vi "VI-Hacker.vi"(8 "error in (no error)":errorcluster, 11 "Path to VI (*.vi, *.vit, *.vim)":path) -> (0 "error out":errorcluster)   [LabVIEW 2022 SP3, in "VI-Hacker.lvlib"]
doc: "Unlocks a password protected VI.\n\nCreated by: Ryan Pacini (c) 2023"
uses:
  VI-Hacker.lvlib
panel:
  # "Unlock a Password Protected VI\nCreated by: Ryan Pacini (c) 2023"
  # "Instructions:\n1. Enter path to password protected VI (*.vi)\n2. Run this VI\nNote: A new VI is created, the original source file remains unmodified."
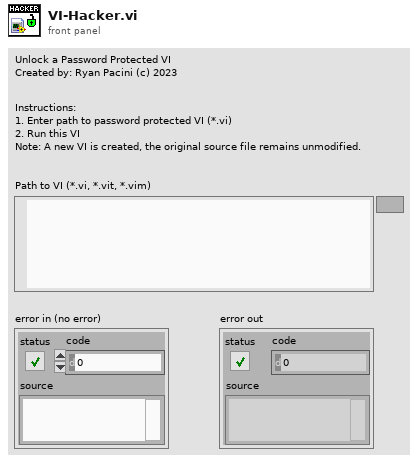
[diagram p1: front panel]
types:
  T1 = cluster{"BLOCK_INFO":cluster{"Int1":u32, "Int2":u32, "Int3":u32, "Offset":u32, "Size":u32}[]}
  T2 = cluster{"Name":string, "Idx":i32, "Data":string, "Offset":u32}
  T3 = enum16{"open", "replace", "create", "open or create", "replace or create", "replace or create with confirmation"}
  T4 = cluster{"vers":i32, "BDPW":i32, "LIBN":i32, "LVSR":i32, "BDHx":i32}
  T5 = cluster{"Version Major":u8, "Pswrd Hashes":cluster{"Pswrd (md5)":string, "Hash1 (md5)":string, "Hash2 (md5)":string}, "Owning Libs (':')":string, "Pswrd Salt (md5)":string, "Diagram (md5)":string, "BDPW Offset":u32, "New BDPW":string}
  T6 = cluster{"Pswrd (md5)":string, "Hash1 (md5)":string, "Hash2 (md5)":string}
  T7 = enum32{"invalid lock state", "Not Locked", "Locked (No Password)", "Password-protected"}
  T8 = cluster{"RSRC_Identifier":u64, "RSRC_Type":u32, "RSRC_Creator":u32, "Info_Offset":u32, "Info_Size":u32, "Data_Offset":u32, "Data_Size":u32}
  T9 = cluster{"Int1":u32, "Int2":u32, "Int3":u32, "Offset":u32, "Size":u32}
  T10 = cluster{"Int1":u32, "Int2":u32, "Int3":u32, "Offset":u32, "Size":u32}[]
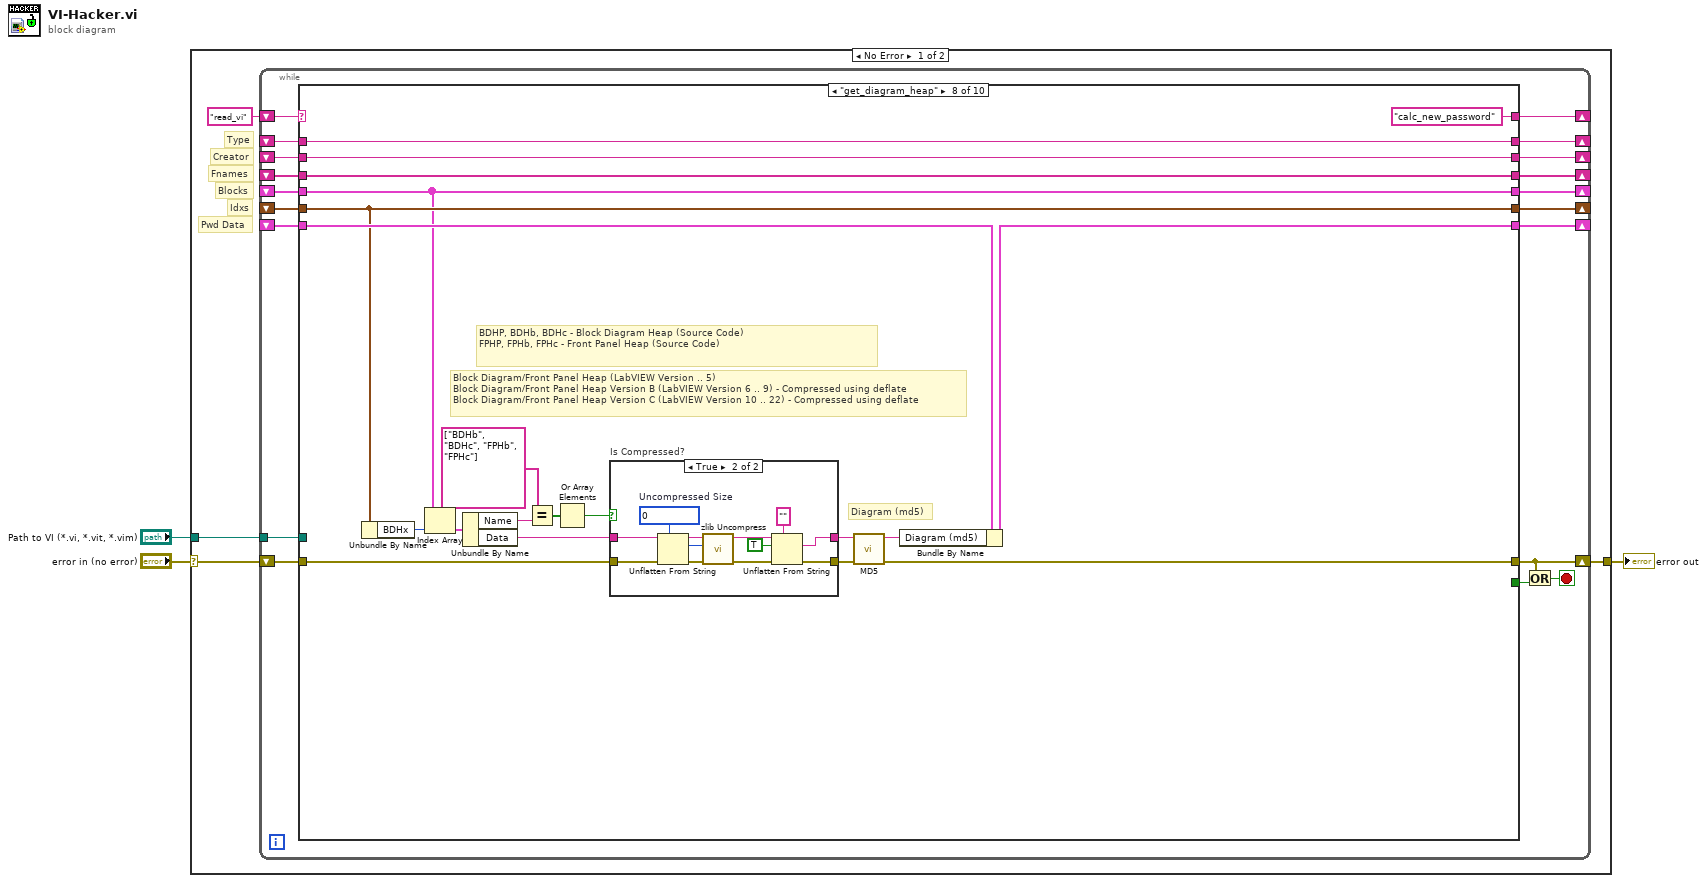
[diagram p0: block diagram]
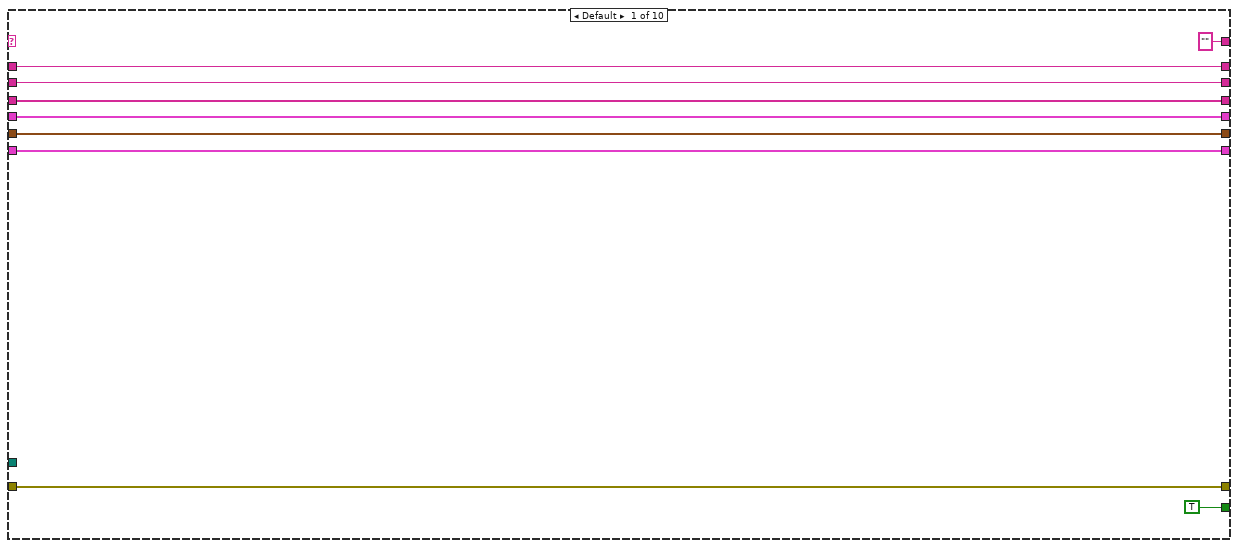
[diagram p2: hidden frame]
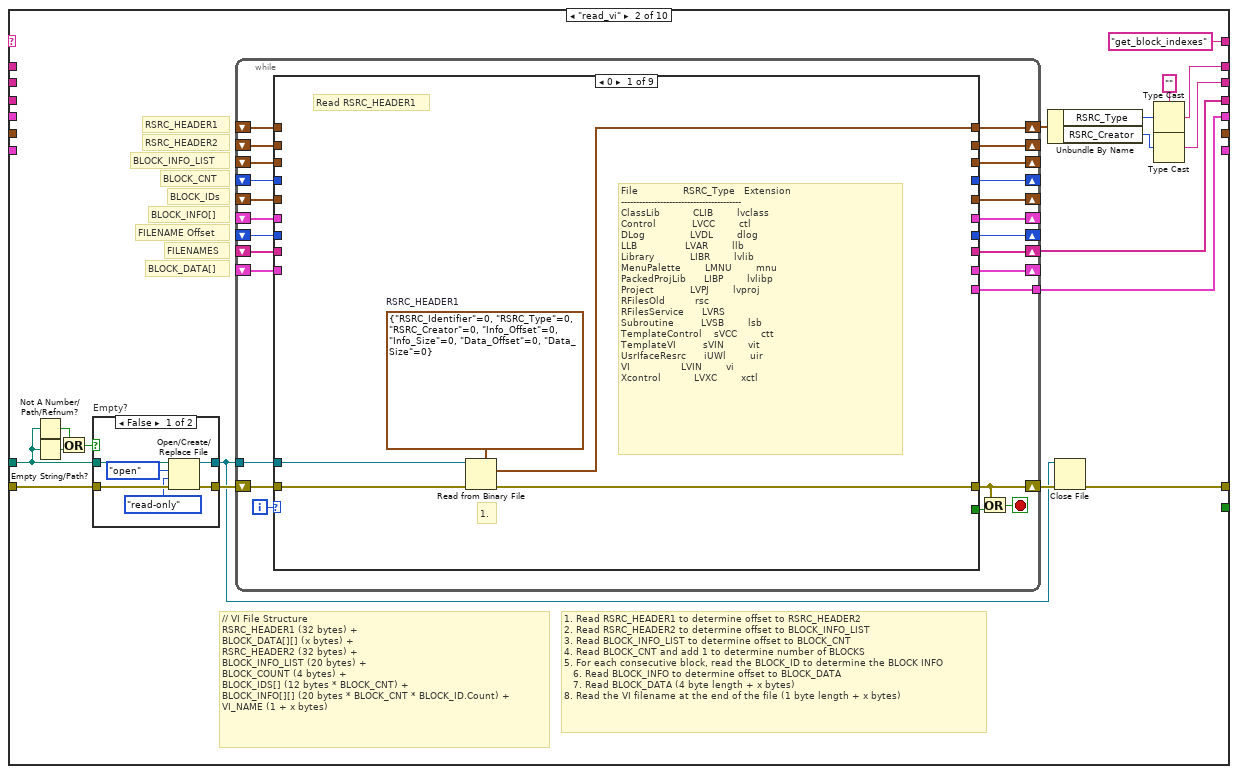
[diagram p3: hidden frame]
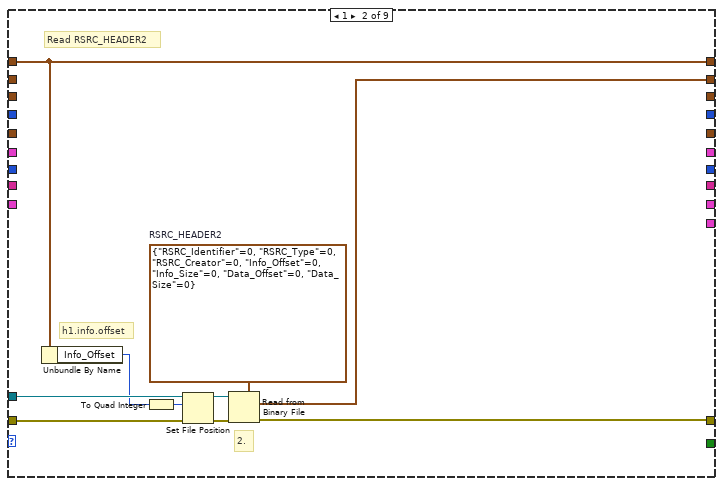
[diagram p4: hidden frame]
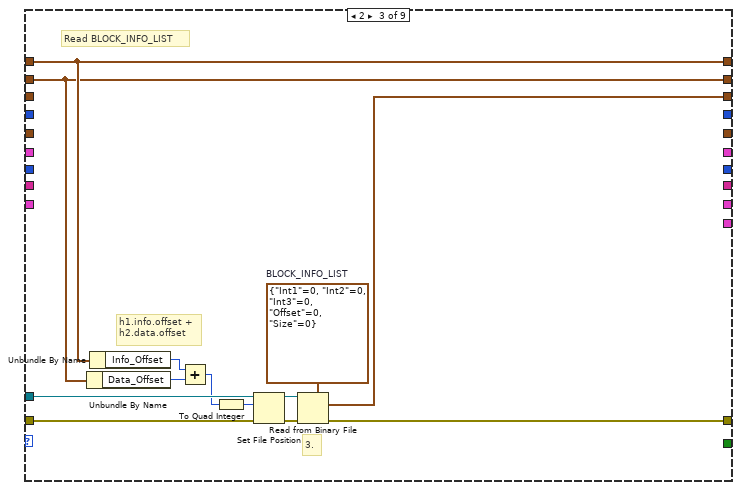
[diagram p5: hidden frame]
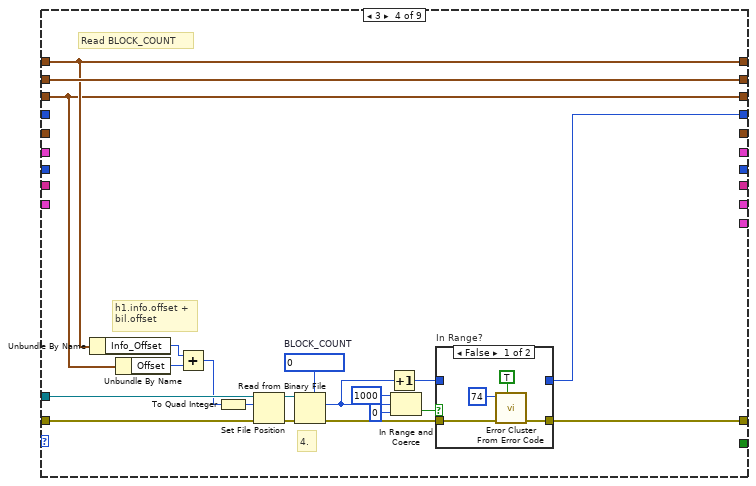
[diagram p6: hidden frame]
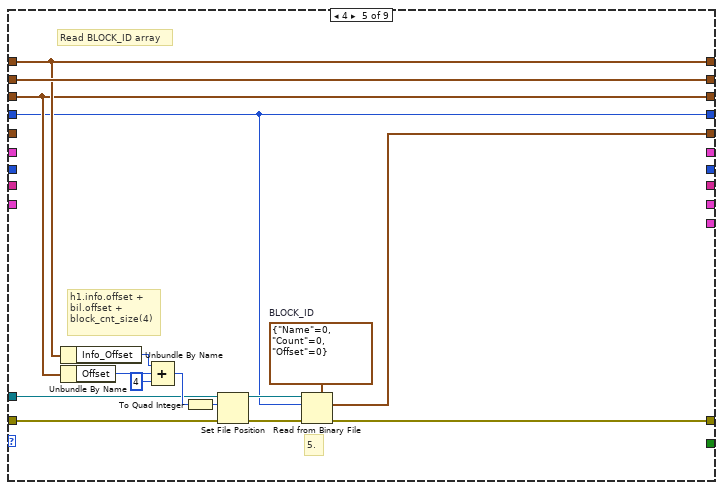
[diagram p8: hidden frame]
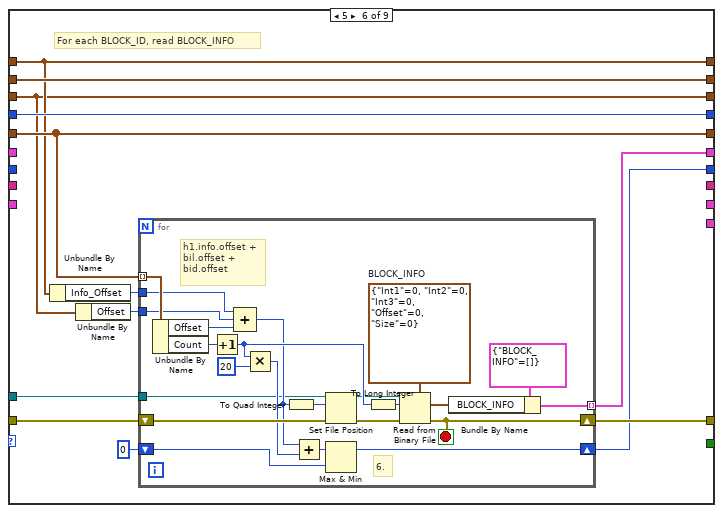
[diagram p9: hidden frame]
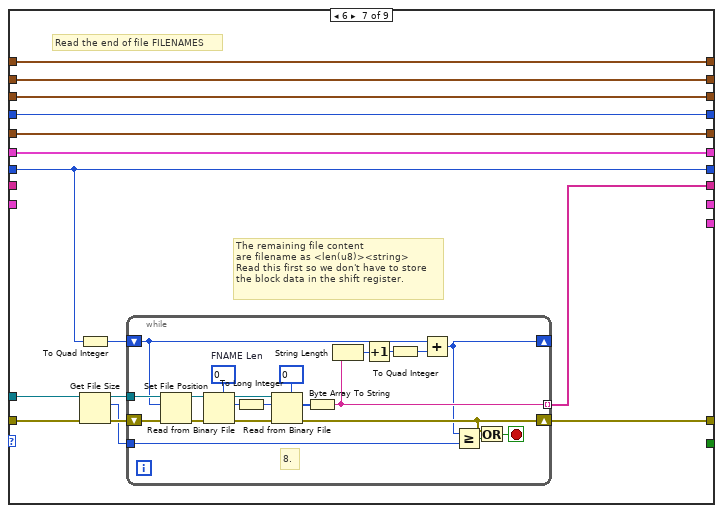
[diagram p10: hidden frame]
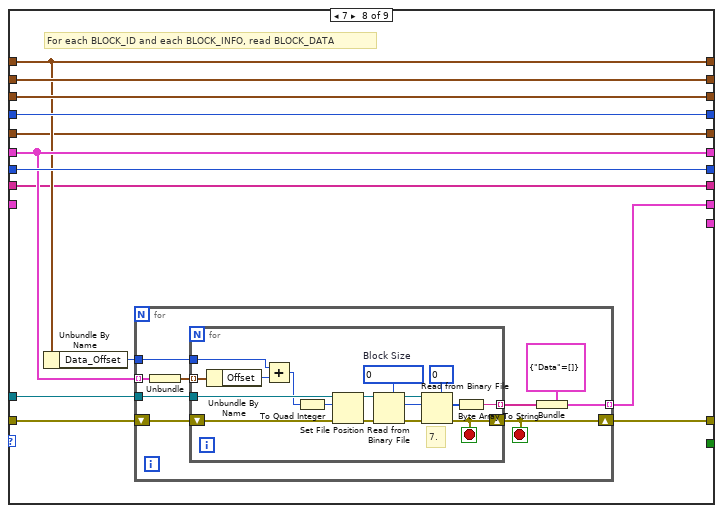
[diagram p11: hidden frame]
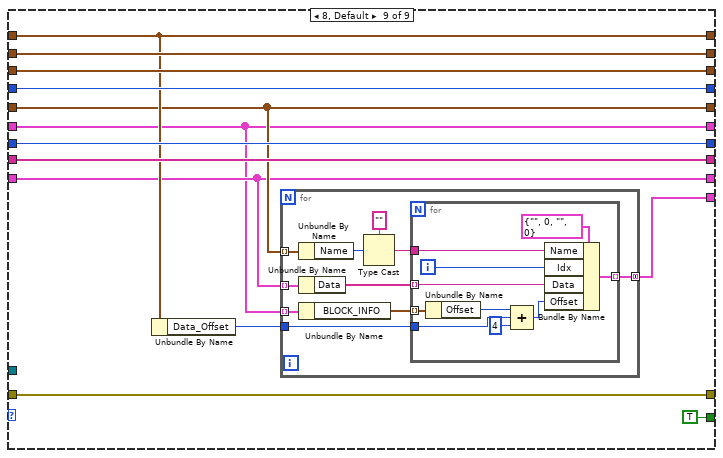
[diagram p12: hidden frame]
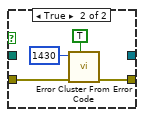
[diagram p13: hidden frame]
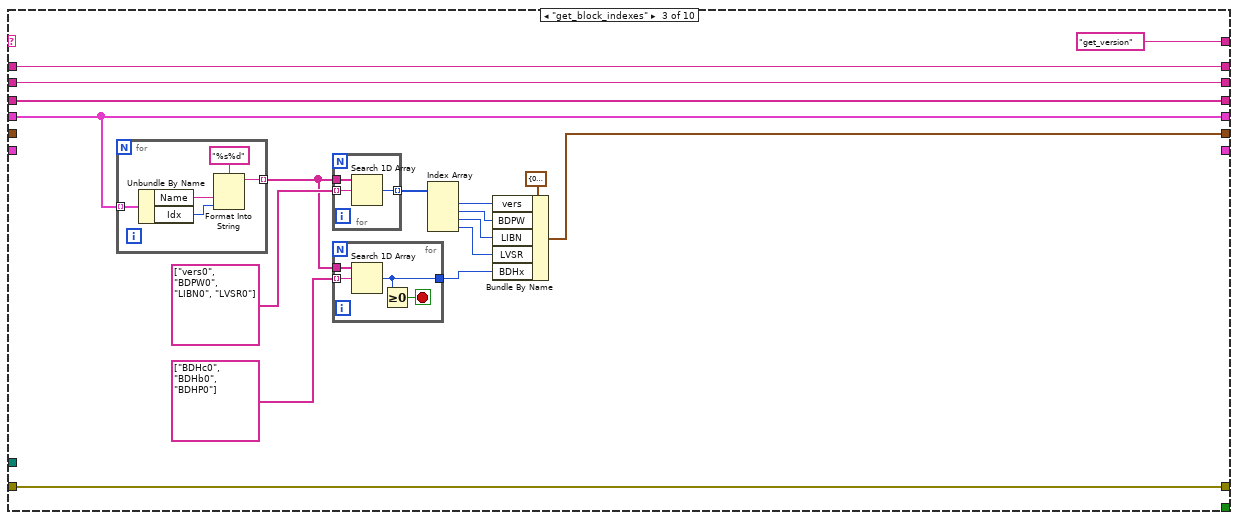
[diagram p14: hidden frame]
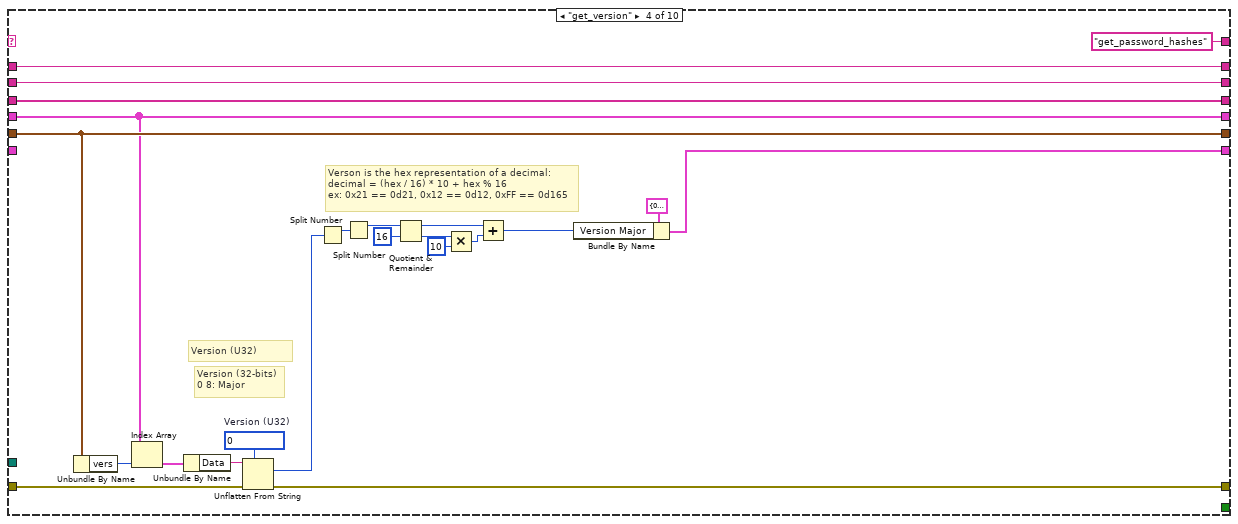
[diagram p15: hidden frame]
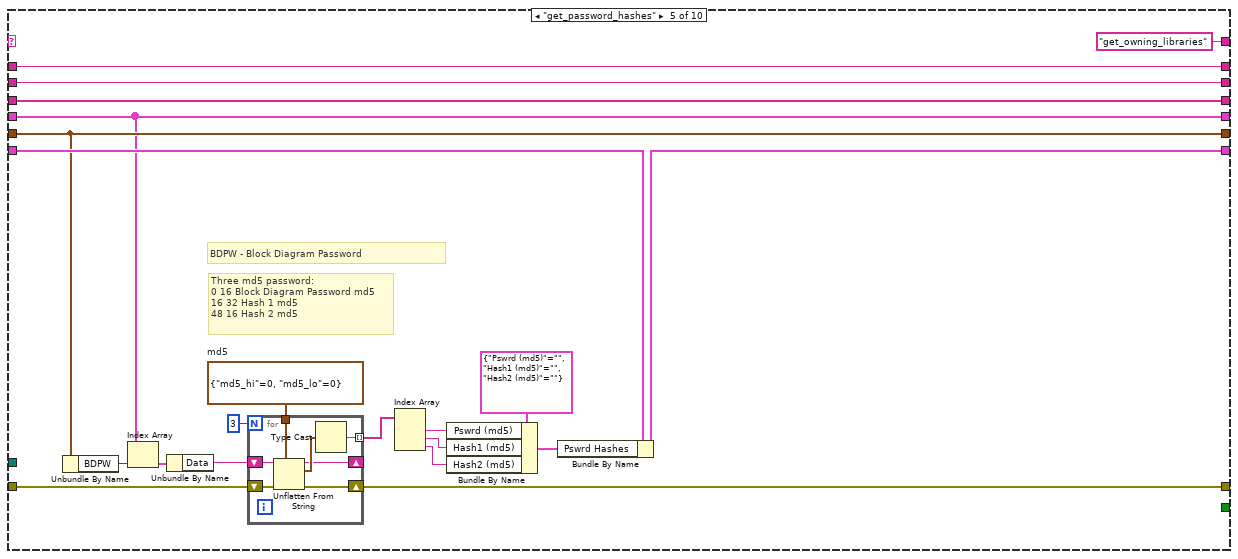
[diagram p16: hidden frame]
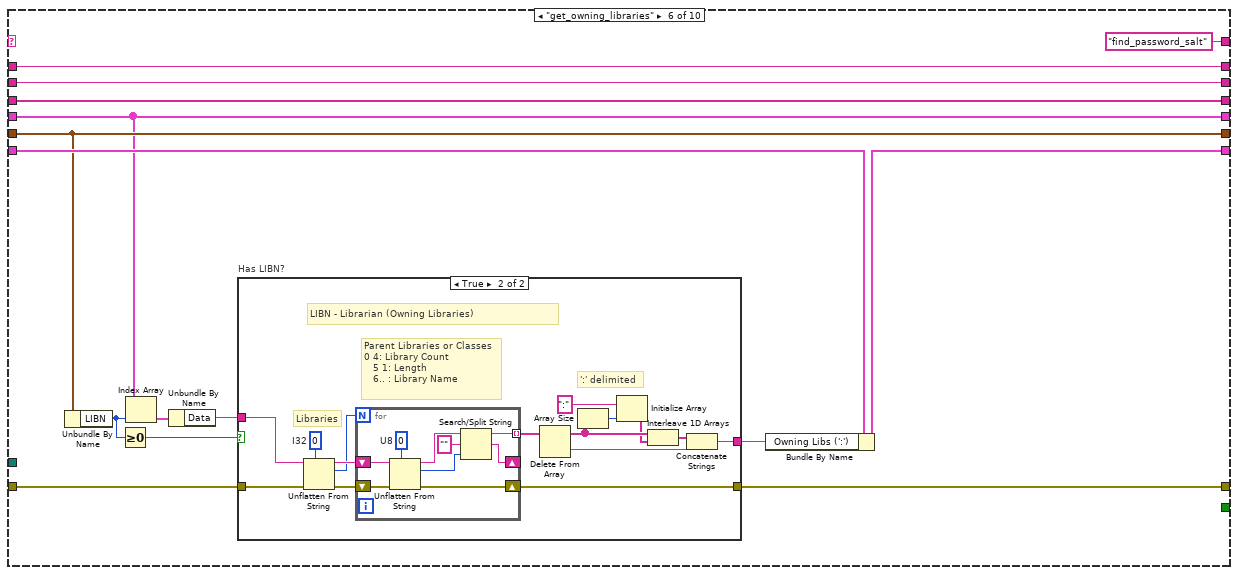
[diagram p17: hidden frame]
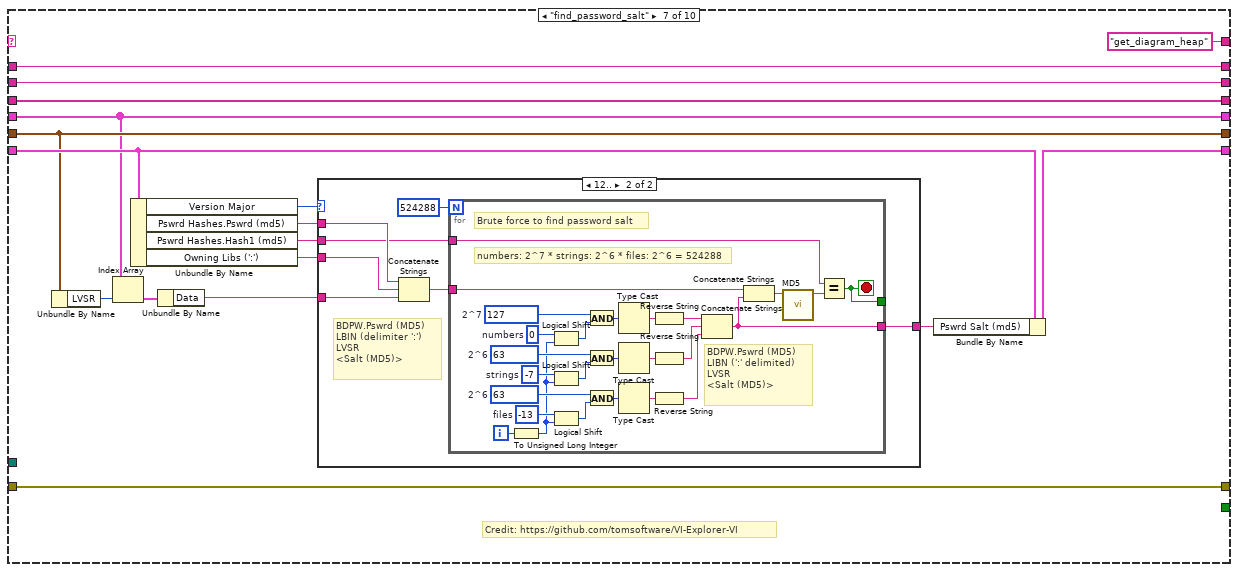
[diagram p19: hidden frame]
diagram:
  n1 = case shown="No Error" "error in (no error)" {
    selector: "error in (no error)" -> [w7 w582]
    tunnel: "Path to VI (*.vi, *.vit, *.vim)" -> [w6 _]
    tunnel: [w5 w582] -> w2
    frame No Error {
      # "Pwd Data"
      # "Idxs"
      # "Blocks"
      # "Fnames"
      # "Creator"
      # "Type"
      n2 = while {
        tunnel: w6 -> [w25]
        shift-right: [w20] -> w5
        shift-left: w7 -> [w26]
        shift-right: [w18] -> _
        shift-left: "read_vi" -> [w21]
        shift-right: [w12] -> _
        shift-left: _ -> [w16]
        shift-right: [w24] -> _
        shift-left: _ -> [w15]
        shift-right: [w22] -> _
        shift-left: _ -> [w14]
        shift-right: [w23] -> _
        shift-left: _ -> [w13]
        shift-right: [w11] -> _
        shift-left: _ -> [w10]
        shift-right: [w9] -> _
        shift-left: _ -> [w8]
        stop <- w19 stop-if-true
        n3 = case shown="\"get_diagram_heap\"" w21 {
          tunnel: w26 -> [w35 w53 w304 w335 w364 w388 w438 w480 w532 w535]
          tunnel: w25 -> [_ w52 _ _ _ _ _ _ _ w540]
          tunnel: [w32 w48 w319 w354 w375 w397 w439 w491 w533 w568] -> w24
          tunnel: [w35 w45 w304 w334 w363 w387 w438 w477 w532 w536] -> w20
          tunnel: [w33 w43 w316 w340 w360 w392 w429 w485 w515 w567] -> w12
          tunnel: [w30 w39 w318 w353 w374 w396 w437 w490 w531 w566] -> w23
          tunnel: [w31 w37 w317 w352 w373 w395 w436 w489 w530 w565] -> w22
          tunnel: ["" "get_block_indexes" "get_version" "get_password_hashes" "get_owning_libraries" "find_password_salt" "get_diagram_heap" "calc_new_password" "new_vi" ""] -> w18
          tunnel: [TRUE _ _ _ _ _ _ _ _ TRUE] -> w17
          tunnel: w16 -> [w33 _ w316 w340 w360 w392 w429 w485 w515 w567]
          tunnel: w15 -> [w32 _ w319 w354 w375 w397 w439 w491 w533 w568]
          tunnel: w14 -> [w31 _ w317 w352 w373 w395 w436 w489 w530 w565]
          tunnel: w13 -> [w30 _ w318 w353 w374 w396 w437 w490 w531 w566]
          tunnel: [w29 _ w305 w342 w362 w393 w431 w487 w517 w564] -> w11
          tunnel: w10 -> [w29 _ _ w342 w362 w393 w431 w487 w517 w564]
          tunnel: [w28 _ _ w333 w357 w390 w426 w475 w509 w539] -> w9
          tunnel: w8 -> [w28 _ _ _ w372 w394 w433 w488 w521 w539]
          frame Default {
          }
          frame "read_vi" {
            w36 = "" ("type")
            # "1. Read RSRC_HEADER1 to determine offset to RSRC_HEADER2\n2. Read RSRC_HEADER2 to determine offset to BLOCK_INFO_LIST\n3. Read BLOCK_INFO_LIST to determine offset to BLOCK_CNT\n4. Read BLOCK_CNT and add 1 to determine number of BLOCKS\n5. For each consecutive block, read the BLOCK_ID to determine the BLOCK INFO\n   6. Read BLOCK_INFO to determine offset to BLOCK_DATA\n   7. Read BLOCK_DATA (4 byte length + x bytes)\n8. Read the VI filename at the end of the file (1 byte length + x bytes)"
            # "// VI File Structure\nRSRC_HEADER1 (32 bytes) + \nBLOCK_DATA[][] (x bytes) +\nRSRC_HEADER2 (32 bytes) + \nBLOCK_INFO_LIST (20 bytes) +\nBLOCK_COUNT (4 bytes) + \nBLOCK_IDS[] (12 bytes * BLOCK_CNT) +\nBLOCK_INFO[][] (20 bytes * BLOCK_CNT * BLOCK_ID.Count) +\nVI_NAME (1 + x bytes)"
            # "BLOCK_DATA[]"
            # "FILENAME Offset"
            # "BLOCK_INFO[]"
            # "BLOCK_IDs"
            # "BLOCK_CNT"
            # "BLOCK_INFO_LIST"
            # "RSRC_HEADER2"
            # "FILENAMES"
            # "RSRC_HEADER1"
            n4 = Not A Number/Path/Refnum?(number/path/refnum=w52) -> (NaN/Path/Refnum?=w50:bool)
            n5 = Empty String/Path?(string/path=w52) -> (empty?=w51:bool)
            n6 = Or(x=w50, y=w51) -> (x .or. y?=w49:bool)
            n7 = case "Empty?" shown="False" w49 {
              tunnel: w53 -> [w298 w302]
              tunnel: w52 -> [w295 _]
              tunnel: [w294 w299] -> w47
              tunnel: [w293 _] -> w44
              frame False {
                n8 = Open/Create/Replace File(file path (use dialog)=w295, error in=w298, operation (0:open)=T3."open", access (0:read/write)=enum16{"read/write", "read-only", "write-only"}."read-only") -> (refnum out=w293:refnum<file>, error out=w294:errorcluster)  [unwired: 2 in, 1 out]
              }
              frame True {
                n9 = call <vilib>:"Error Cluster From Error Code.vi"("show call chain? (False)"=TRUE, "error in (no error)"=w302, "error code (0)"=1430) -> ("error out"=w299:errorcluster)  [unwired: 6 in]
              }
            }
            n10 = while {
              tunnel: w44 -> [w77]
              shift-right: [w73] -> w46
              shift-left: w47 -> [w78]
              shift-right: [w75] -> w42
              shift-left: _ -> [w74]
              shift-right: [w70] -> _
              shift-left: _ -> [w69]
              shift-right: [w68] -> _
              shift-left: _ -> [w67]
              shift-right: [w66] -> _
              shift-left: _ -> [w65]
              shift-right: [w64] -> _
              shift-left: _ -> [w63]
              shift-right: [w62] -> _
              shift-left: _ -> [w61]
              shift-right: [w60] -> _
              shift-left: _ -> [w59]
              shift-right: [w57] -> w48
              shift-left: _ -> [w56]
              shift-right: [w58] -> _
              shift-left: _ -> [w55]
              tunnel: [w54] -> w43
              i -> [w76]
              stop <- w72 stop-if-true
              n11 = case shown="0" w76 {
                tunnel: w78 -> [w83 w93 w106 w122 w145 w159 w193 w229 w266]
                tunnel: [w81 w91 w105 w121 w144 w157 w192 w223 w266] -> w73
                tunnel: w77 -> [w82 w88 w98 w111 w136 w158 w189 w225 _]
                tunnel: [w79 w92 w104 w120 w143 w155 w199 w227 w265] -> w75
                tunnel: w74 -> [_ w92 w104 w120 w143 w155 w199 w227 w265]
                tunnel: [_ _ _ _ _ _ _ _ TRUE] -> w71
                tunnel: [_ w90 w103 w126 w148 w161 w198 w233 w272] -> w70
                tunnel: w69 -> [_ _ w103 w126 w148 w161 w198 w233 w272]
                tunnel: [_ _ w100 w119 w142 w154 w197 w232 w271] -> w68
                tunnel: w67 -> [_ _ _ w119 w142 w154 w197 w232 w271]
                tunnel: [_ _ _ w113 w134 w160 w196 w231 w270] -> w66
                tunnel: w65 -> [_ _ _ _ w134 w160 w196 w231 w270]
                tunnel: [_ _ _ _ w133 w156 w195 w224 w264] -> w64
                tunnel: w63 -> [_ _ _ _ _ w156 w195 w224 w264]
                tunnel: [_ _ _ _ _ w150 w194 w228 w261] -> w62
                tunnel: w61 -> [_ _ _ _ _ _ w194 w228 w261]
                tunnel: [_ _ _ _ _ w149 w187 w230 w269] -> w60
                tunnel: w59 -> [_ _ _ _ _ _ w187 w230 w269]
                tunnel: [_ _ _ _ _ _ _ w222 w263] -> w58
                tunnel: [_ _ _ _ _ _ w191 w221 w268] -> w57
                tunnel: w56 -> [_ _ _ _ _ _ _ w221 w268]
                tunnel: w55 -> [_ _ _ _ _ _ _ _ w263]
                tunnel: [_ _ _ _ _ _ _ _ w262] -> w54
                frame 0 {
                  w80 = T8 {"RSRC_Identifier"=0, "RSRC_Type"=0, "RSRC_Creator"=0, "Info_Offset"=0, "Info_Size"=0, "Data_Offset"=0, "Data_Size"=0}  # RSRC_HEADER1
                  # "File               RSRC_Type   Extension\n----------------------------------------\nClassLib           CLIB        lvclass\nControl            LVCC        ctl\nDLog               LVDL        dlog\nLLB                LVAR        llb\nLibrary            LIBR        lvlib\nMenuPalette        LMNU        mnu\nPackedProjLib      LIBP        lvlibp\nProject            LVPJ        lvproj\nRFilesOld          rsc         \nRFilesService      LVRS        \nSubroutine         LVSB        lsb\nTemplateControl    sVCC        ctt\nTemplateVI         sVIN        vit\nUsrIfaceResrc      iUWl        uir\nVI                 LVIN        vi\nXcontrol           LVXC        xctl"
                  # "Read RSRC_HEADER1"
                  # "1."
                  n12 = Read from Binary File(5:w80, 8:w83, 11:w82) -> (0:w81:errorcluster, 2:w79:T8)  [unwired: 3 in, 2 out]
                }
                frame 1 {
                  w86 = T8 {"RSRC_Identifier"=0, "RSRC_Type"=0, "RSRC_Creator"=0, "Info_Offset"=0, "Info_Size"=0, "Data_Offset"=0, "Data_Size"=0}  # RSRC_HEADER2
                  # "Read RSRC_HEADER2"
                  # "2."
                  # "h1.info.offset"
                  n13 = Unbundle By Name(w92) -> ("Info_Offset"=w87:u32)
                  n14 = To Quad Integer(1:w87) -> (0:w84:i64)
                  n15 = Set File Position(offset (in bytes) (0)=w84, refnum=w88, error in=w93) -> (refnum out=w85:refnum<file>, error out=w89:errorcluster)  [unwired: 1 in]
                  n16 = Read from Binary File(5:w86, 8:w89, 11:w85) -> (0:w91:errorcluster, 2:w90:T8)  [unwired: 3 in, 2 out]
                }
                frame 2 {
                  w97 = T9 {"Int1"=0, "Int2"=0, "Int3"=0, "Offset"=0, "Size"=0}  # BLOCK_INFO_LIST
                  # "Read BLOCK_INFO_LIST"
                  # "3."
                  # "h1.info.offset +\nh2.data.offset"
                  n17 = Unbundle By Name(w103) -> ("Data_Offset"=w102:u32)
                  n18 = Unbundle By Name(w104) -> ("Info_Offset"=w101:u32)
                  n19 = Add(x=w101, y=w102) -> (x+y=w95:u32)
                  n20 = To Quad Integer(1:w95) -> (0:w94:i64)
                  n21 = Set File Position(offset (in bytes) (0)=w94, refnum=w98, error in=w106) -> (refnum out=w96:refnum<file>, error out=w99:errorcluster)  [unwired: 1 in]
                  n22 = Read from Binary File(5:w97, 8:w99, 11:w96) -> (0:w105:errorcluster, 2:w100:T9)  [unwired: 3 in, 2 out]
                }
                frame 3 {
                  w110 = 0  # BLOCK_COUNT
                  # "Read BLOCK_COUNT"
                  # "4."
                  # "h1.info.offset +\nbil.offset"
                  n23 = Unbundle By Name(w120) -> ("Info_Offset"=w117:u32)
                  n24 = Unbundle By Name(w119) -> ("Offset"=w118:u32)
                  n25 = Add(x=w117, y=w118) -> (x+y=w108:u32)
                  n26 = To Quad Integer(1:w108) -> (0:w107:i64)
                  n27 = Set File Position(offset (in bytes) (0)=w107, refnum=w111, error in=w122) -> (refnum out=w109:refnum<file>, error out=w112:errorcluster)  [unwired: 1 in]
                  n28 = Read from Binary File(5:w110, 8:w112, 11:w109) -> (0:w123:errorcluster, 2:w114:i32)  [unwired: 3 in, 2 out]
                  n29 = Increment(x=w114) -> (x+1=w115:i32)
                  n30 = In Range and Coerce(upper limit=1000, x=w114, lower limit=0) -> (In Range?=w116:bool)  [unwired: 1 out]
                  n31 = case "In Range?" shown="False" w116 {
                    tunnel: w123 -> [w128 w132]
                    tunnel: [w127 w132] -> w121
                    tunnel: w115 -> [_ w131]
                    tunnel: [_ w131] -> w113
                    frame False {
                      n32 = call <vilib>:"Error Cluster From Error Code.vi"("show call chain? (False)"=TRUE, "error in (no error)"=w128, "error code (0)"=74) -> ("error out"=w127:errorcluster)  [unwired: 6 in]
                    }
                    frame True {
                    }
                  }
                }
                frame 4 {
                  w138 = cluster{"Name":u32, "Count":u32, "Offset":u32} {"Name"=0, "Count"=0, "Offset"=0}  # BLOCK_ID
                  # "Read BLOCK_ID array"
                  # "5."
                  # "h1.info.offset +\nbil.offset +\nblock_cnt_size(4)"
                  n33 = Unbundle By Name(w143) -> ("Info_Offset"=w147:u32)
                  n34 = Unbundle By Name(w142) -> ("Offset"=w146:u32)
                  n35 = Compound Arithmetic op=ADD(w147, w146, u32 4 ("value")) -> (w137:u32)
                  n36 = To Quad Integer(1:w137) -> (0:w135:i64)
                  n37 = Set File Position(offset (in bytes) (0)=w135, refnum=w136, error in=w145) -> (refnum out=w139:refnum<file>, error out=w140:errorcluster)  [unwired: 1 in]
                  n38 = Read from Binary File(5:w138, 8:w140, 10:w134, 11:w139) -> (0:w144:errorcluster, 2:w133:cluster{"Name":u32, "Count":u32, "Offset":u32}[])  [unwired: 2 in, 2 out]
                }
                frame 5 {
                  # "For each BLOCK_ID, read BLOCK_INFO"
                  n39 = Unbundle By Name(w155) -> ("Info_Offset"=w153:u32)
                  n40 = Unbundle By Name(w154) -> ("Offset"=w152:u32)
                  n41 = for {
                    tunnel: w158 -> [w164]
                    shift-right: [w171] -> w157
                    shift-left: w159 -> [w184]
                    tunnel: w156 -> [w183] mode=indexing
                    tunnel: w153 -> [w179]
                    tunnel: w152 -> [w178]
                    shift-right: [w175] -> w149
                    shift-left: u32 0 -> [w174]
                    tunnel: [w172] -> w150 mode=indexing
                    stop <- w171 stop-if-true
                    w170 = T9 {"Int1"=0, "Int2"=0, "Int3"=0, "Offset"=0, "Size"=0}  # BLOCK_INFO
                    # "6."
                    # "h1.info.offset +\nbil.offset +\nbid.offset"
                    n42 = Unbundle By Name(w183) -> ("Offset"=w180:u32, "Count"=w181:u32)
                    n43 = Increment(x=w181) -> (x+1=w169:u32)
                    n44 = Compound Arithmetic op=ADD(w179, w178, w180) -> (w165:u32)
                    n45 = Multiply(x=w169, y=u32 20 ("length (rest)")) -> (x*y=w177:u32)
                    n46 = To Quad Integer(1:w165) -> (0:w163:i64)
                    n47 = Add(x=w165, y=w177) -> (x+y=w176:u32)
                    n48 = Set File Position(offset (in bytes) (0)=w163, refnum=w164, error in=w184) -> (refnum out=w167:refnum<file>, error out=w168:errorcluster)  [unwired: 1 in]
                    n49 = Max & Min(x=w176, y=w174) -> (max(x,y)=w175:u32)  [unwired: 1 out]
                    n50 = To Long Integer(number=w169) -> (32bit integer=w166:i32)
                    n51 = Read from Binary File(5:w170, 8:w168, 10:w166, 11:w167) -> (0:w171:errorcluster, 2:w173:T10)  [unwired: 2 in, 2 out]
                    n52 = Bundle By Name(cluster=T1 {"BLOCK_INFO"=[]}, "BLOCK_INFO"=w173) -> (w172:T1)
                  }
                }
                frame 6 {
                  # "Read the end of file FILENAMES"
                  # "The remaining file content\nare filename as <len(u8)><string>\nRead this first so we don't have to store\nthe block data in the shift register."
                  n53 = To Quad Integer(1:w187) -> (0:w186:i64)
                  n54 = Get File Size(file=w189, error in=w193) -> (refnum out=w188:refnum<file>, size (in bytes)=w185:i64, 0:w190:errorcluster)
                  n55 = while {
                    tunnel: [w209] -> w191 mode=indexing
                    tunnel: w188 -> [w218]
                    shift-right: [w207] -> w192
                    shift-left: w190 -> [w220]
                    shift-right: [w202] -> _
                    shift-left: w186 -> [w203]
                    tunnel: w185 -> [w201]
                    stop <- w206 stop-if-true
                    w215 = u8 0  # FNAME Len
                    # "8."
                    n56 = Set File Position(offset (in bytes) (0)=w203, refnum=w218, error in=w220) -> (refnum out=w217:refnum<file>, error out=w219:errorcluster)  [unwired: 1 in]
                    n57 = Read from Binary File(5:w215, 8:w219, 11:w217) -> (0:w216:errorcluster, 2:w212:u8, 3:w213:refnum<file>)  [unwired: 3 in, 1 out]
                    n58 = To Long Integer(number=w212) -> (32bit integer=w211:i32)
                    n59 = Read from Binary File(5:u8 0, 8:w216, 10:w211, 11:w213) -> (0:w207:errorcluster, 2:w210:u8[])  [unwired: 2 in, 2 out]
                    n60 = Byte Array To String(unsigned byte array=w210) -> (string=w209:string)
                    n61 = String Length(string=w209) -> (length=w208:i32)
                    n62 = Increment(x=w208) -> (x+1=w205:i32)
                    n63 = To Quad Integer(1:w205) -> (0:w204:i64)
                    n64 = Add(x=w203, y=w204) -> (x+y=w202:i64)
                    n65 = Greater Or Equal?(x=w202, y=w201) -> (x >= y?=w200:bool)
                    n66 = Or(x=w207, y=w200) -> (x .or. y?=w206:bool)
                  }
                }
                frame 7 {
                  # "For each BLOCK_ID and each BLOCK_INFO, read BLOCK_DATA"
                  n67 = Unbundle By Name(w227) -> ("Data_Offset"=w226:u32)
                  n68 = for {
                    tunnel: w228 -> [w241] mode=indexing
                    tunnel: w226 -> [w239]
                    tunnel: w225 -> [w238]
                    shift-right: [w237] -> w223
                    shift-left: w229 -> [w242]
                    tunnel: [w235] -> w222 mode=indexing
                    stop <- w237 stop-if-true
                    n69 = Unbundle(w241) -> ("BLOCK_INFO"=w240:T10)
                    n70 = for {
                      tunnel: w238 -> [w252]
                      shift-right: [w254] -> w237
                      shift-left: w242 -> [w259]
                      tunnel: [w243] -> w236 mode=indexing
                      tunnel: w240 -> [w256] mode=indexing
                      tunnel: w239 -> [w255]
                      stop <- w254 stop-if-true
                      w246 = 0  # Block Size
                      # "7."
                      n71 = Unbundle By Name(w256) -> ("Offset"=w258:u32)
                      n72 = Add(x=w255, y=w258) -> (x+y=w251:u32)
                      n73 = To Quad Integer(1:w251) -> (0:w250:i64)
                      n74 = Set File Position(offset (in bytes) (0)=w250, refnum=w252, error in=w259) -> (refnum out=w248:refnum<file>, error out=w253:errorcluster)  [unwired: 1 in]
                      n75 = Read from Binary File(5:w246, 8:w253, 11:w248) -> (0:w249:errorcluster, 2:w244:i32, 3:w247:refnum<file>)  [unwired: 3 in, 1 out]
                      n76 = Read from Binary File(5:u8 0, 8:w249, 10:w244, 11:w247) -> (0:w254:errorcluster, 2:w257:u8[])  [unwired: 2 in, 2 out]
                      n77 = Byte Array To String(unsigned byte array=w257) -> (string=w243:string)
                    }
                    n78 = Bundle(cluster=cluster{"Data":string[]} {"Data"=[]}, "Data"=w236) -> (w235:cluster{"Data":string[]})
                  }
                }
                frame 8, Default {
                  n79 = Unbundle By Name(w265) -> ("Data_Offset"=w260:u32)
                  n80 = for {
                    tunnel: w264 -> [w282] mode=indexing
                    tunnel: [w273] -> w262 mode=concatenating
                    tunnel: w263 -> [w279] mode=indexing
                    tunnel: w261 -> [w278] mode=indexing
                    tunnel: w260 -> [w276]
                    n81 = Unbundle By Name(w282) -> ("Name"=w281:u32)
                    n82 = Unbundle By Name(w279) -> ("Data"=w275:string[])
                    n83 = Unbundle By Name(w278) -> ("BLOCK_INFO"=w277:T10)
                    n84 = Type Cast(type="", x=w281) -> (*(type *) &x=w274:string)
                    n85 = for {
                      tunnel: w277 -> [w292] mode=indexing
                      tunnel: w276 -> [w290]
                      tunnel: w275 -> [w285] mode=indexing
                      tunnel: w274 -> [w287]
                      tunnel: [w283] -> w273 mode=indexing
                      i -> [w286]
                      n86 = Unbundle By Name(w292) -> ("Offset"=w289:u32)
                      n87 = Compound Arithmetic op=ADD(w289, w290, u32 4 ("value")) -> (w284:u32)
                      n88 = Bundle By Name(cluster=T2 {"Name"="", "Idx"=0, "Data"="", "Offset"=0} ("Block"), "Name"=w287, "Idx"=w286, "Data"=w285, "Offset"=w284) -> (w283:T2)
                    }
                  }
                }
              }
              n89 = Or(x=w73, y=w71) -> (x .or. y?=w72:bool)
            }
            n90 = Unbundle By Name(w42) -> ("RSRC_Type"=w41:u32, "RSRC_Creator"=w40:u32)
            n91 = Close File(refnum=w44, error in=w46) -> (error out=w45:errorcluster)  [unwired: 1 out]
            n92 = Type Cast(type=w36, x=w41) -> (*(type *) &x=w39:string)
            n93 = Type Cast(type=w36, x=w40) -> (*(type *) &x=w37:string)
          }
          frame "get_block_indexes" {
            n94 = for {
              tunnel: w316 -> [w331] mode=indexing
              tunnel: [w327] -> w308 mode=indexing
              n95 = Unbundle By Name(w331) -> ("Name"=w330:string, "Idx"=w328:i32)
              n96 = Format Into String(format string="%s%d", w330, w328) -> (resulting string=w327:string)  [unwired: 2 in, 1 out]
            }
            n97 = for {
              tunnel: w308 -> [w326]
              tunnel: string[] ["vers0", "BDPW0", "LIBN0", "LVSR0"] -> [w325] mode=indexing
              tunnel: [w324] -> w314 mode=indexing
              n98 = Search 1D Array(1D array=w326, element=w325) -> (index of element=w324:i32)  [unwired: 1 in]
            }
            n99 = for {
              tunnel: w308 -> [w323]
              tunnel: string[] ["BDHc0", "BDHb0", "BDHP0"] -> [w322] mode=indexing
              tunnel: [w321] -> w306
              stop <- w320 stop-if-true
              n100 = Search 1D Array(1D array=w323, element=w322) -> (index of element=w321:i32)  [unwired: 1 in]
              n101 = Greater Or Equal To 0?(x=w321) -> (x >= 0?=w320:bool)
            }
            n102 = Index Array(array=w314) -> (element #1=w312:i32, element #2=w311:i32, element #3=w310:i32, element #4=w309:i32)  [unwired: 4 in]
            n103 = Bundle By Name(cluster=T4 {"vers"=0, "BDPW"=0, "LIBN"=0, "LVSR"=0, "BDHx"=0} ("Block Idxs"), "vers"=w312, "BDPW"=w311, "LIBN"=w310, "LVSR"=w309, "BDHx"=w306) -> (w305:T4)
          }
          frame "get_version" {
            w344 = u32 0  # Version (U32)
            # "Version (U32)"
            # "Verson is the hex representation of a decimal:\ndecimal = (hex / 16) * 10 + hex % 16\nex: 0x21 == 0d21, 0x12 == 0d12, 0xFF == 0d165"
            # "Version (32-bits)\n0 8: Major"
            n104 = Unbundle By Name(w342) -> ("vers"=w341:i32)
            n105 = Index Array(array=w340, index=w341) -> (element=w339:T2)
            n106 = Unbundle By Name(w339) -> ("Data"=w338:string)
            n107 = Unflatten From String(type=w344, binary string=w338, error in (no error)=w335) -> (value=w343:u32, error out=w334:errorcluster)  [unwired: 2 in, 1 out]
            n108 = Split Number(x=w343) -> (hi(x)=w351:u16)  [unwired: 1 out]
            n109 = Split Number(x=w351) -> (hi(x)=w350:u8)  [unwired: 1 out]
            n110 = Quotient & Remainder(x=w350, y=u8 16) -> (x-y*floor(x/y)=w345:u8, floor(x/y)=w348:u8)
            n111 = Multiply(x=w348, y=u8 10) -> (x*y=w346:u8)
            n112 = Add(x=w345, y=w346) -> (x+y=w336:u8)
            n113 = Bundle By Name(cluster=T5 {"Version Major"=0, "Pswrd Hashes"={"Pswrd (md5)"="", "Hash1 (md5)"="", "Hash2 (md5)"=""}, "Owning Libs (':')"="", "Pswrd Salt (md5)"="", "Diagram (md5)"="", "BDPW Offset"=0, "New BDPW"=""} ("Pwd"), "Version Major"=w336) -> (w333:T5)
          }
          frame "get_password_hashes" {
            w366 = cluster{"md5_hi":u64, "md5_lo":u64} {"md5_hi"=0, "md5_lo"=0}  # md5
            # "BDPW - Block Diagram Password"
            # "Three md5 password:\n0 16 Block Diagram Password md5\n16 32 Hash 1 md5\n48 16 Hash 2 md5"
            n114 = Unbundle By Name(w362) -> ("BDPW"=w361:i32)
            n115 = Index Array(array=w360, index=w361) -> (element=w359:T2)
            n116 = Unbundle By Name(w359) -> ("Data"=w358:string)
            n117 = for {
              N: 3 -> [_]
              shift-right: [w382] -> w363
              shift-left: w364 -> [w381]
              tunnel: [w378] -> w370 mode=indexing
              shift-right: [w377] -> _
              shift-left: w358 -> [w380]
              tunnel: w366 -> [w376]
              n118 = Unflatten From String(type=w376, binary string=w380, error in (no error)=w381) -> (rest of the binary string=w377:string, value=w379:cluster{"md5_hi":u64, "md5_lo":u64}, error out=w382:errorcluster)  [unwired: 2 in]
              n119 = Type Cast(x=w379) -> (*(type *) &x=w378:string)  [unwired: 1 in]
            }
            n120 = Index Array(array=w370) -> (element #1=w369:string, element #2=w368:string, element #3=w367:string)  [unwired: 3 in]
            n121 = Bundle By Name(cluster=T6 {"Pswrd (md5)"="", "Hash1 (md5)"="", "Hash2 (md5)"=""} ("BDPW"), "Pswrd (md5)"=w369, "Hash1 (md5)"=w368, "Hash2 (md5)"=w367) -> (w356:T6)
            n122 = Bundle By Name(cluster=w372, "Pswrd Hashes"=w356) -> (w357:T5)
          }
          frame "get_owning_libraries" {
            n123 = Unbundle By Name(w393) -> ("LIBN"=w384:i32)
            n124 = Greater Or Equal To 0?(x=w384) -> (x >= 0?=w383:bool)
            n125 = Index Array(array=w392, index=w384) -> (element=w391:T2)
            n126 = Unbundle By Name(w391) -> ("Data"=w386:string)
            n127 = case "Has LIBN?" shown="True" w383 {
              tunnel: w388 -> [w398 w402]
              tunnel: [w398 w401] -> w387
              tunnel: w386 -> [_ w400]
              tunnel: [_ w399] -> w385
              frame False {
              }
              frame True {
                w413 = 0  # I32
                # "':' delimited"
                # "LIBN - Librarian (Owning Libraries)"
                # "Parent Libraries or Classes\n0 4: Library Count\n   5 1: Length\n   6.. : Library Name"
                # "Libraries"
                n128 = Unflatten From String(type=w413, binary string=w400, error in (no error)=w402) -> (rest of the binary string=w411:string, value=w410:i32, error out=w412:errorcluster)  [unwired: 2 in]
                n129 = for {
                  N: w410 -> [_]
                  shift-right: [w415] -> _
                  shift-left: w411 -> [w420]
                  shift-right: [w416] -> w401
                  shift-left: w412 -> [w421]
                  tunnel: [w414] -> w403 mode=indexing
                  w422 = u8 0  # U8
                  n130 = Unflatten From String(type=w422, binary string=w420, error in (no error)=w421) -> (rest of the binary string=w419:string, value=w418:u8, error out=w416:errorcluster)  [unwired: 2 in]
                  n131 = Search/Split String(string=w419, search string/char (-)="", offset (0)=w418) -> (substring before match=w414:string, match + rest of string=w415:string)  [unwired: 1 out]
                }
                n132 = Delete From Array(array=w403) -> (deleted portion=w404:string, array with subset deleted=w407:string[])  [unwired: 2 in]
                n133 = Array Size(array=w407) -> (size(s)=w409:i32)
                n134 = Initialize Array(":", w409) -> (w406:string[])
                n135 = Interleave 1D Arrays(w407, w406) -> (w405:string[])
                n136 = Concatenate Strings(w405, w404) -> (w399:string)
              }
            }
            n137 = Bundle By Name(cluster=w394, "Owning Libs (':')"=w385) -> (w390:T5)
          }
          frame "find_password_salt" {
            # "Credit: https://github.com/tomsoftware/VI-Explorer-VI"
            n138 = Unbundle By Name(w431) -> ("LVSR"=w430:i32)
            n139 = Index Array(array=w429, index=w430) -> (element=w428:T2)
            n140 = Unbundle By Name(w433) -> ("Version Major"=w425:u8, "Pswrd Hashes.Pswrd (md5)"=w435:string, "Pswrd Hashes.Hash1 (md5)"=w434:string, "Owning Libs (':')"=w432:string)
            n141 = Unbundle By Name(w428) -> ("Data"=w427:string)
            n142 = case shown="12.." w425 {
              tunnel: w435 -> [_ w444]
              tunnel: w434 -> [_ w443]
              tunnel: w432 -> [_ w442]
              tunnel: w427 -> [_ w441]
              tunnel: [_ w440] -> w424
              frame ..11 {
              }
              frame 12.. {
                # "BDPW.Pswrd (MD5)\nLBIN (delimiter ':')\nLVSR\n<Salt (MD5)>"
                n143 = Concatenate Strings(w444, w442, w441) -> (w445:string)
                n144 = for {
                  N: 524288 -> [_]
                  tunnel: w445 -> [w472]
                  tunnel: w443 -> [w471]
                  tunnel: [w462] -> _
                  tunnel: [w449] -> w440
                  i -> [w467]
                  stop <- w462 stop-if-true
                  w460 = u32 63  # 2^6
                  w461 = u32 63  # 2^6
                  w464 = i8 -13  # files
                  w465 = i8 -7  # strings
                  w466 = i8 0  # numbers
                  w463 = u32 127  # 2^7
                  # "numbers: 2^7 * strings: 2^6 * files: 2^6 = 524288"
                  # "BDPW.Pswrd (MD5)\nLIBN (':' delimited)\nLVSR\n<Salt (MD5)>"
                  # "Brute force to find password salt"
                  n145 = To Unsigned Long Integer(number=w467) -> (unsigned 32bit integer=w459:u32)
                  n146 = Logical Shift(y=w466, x=w459) -> (x << y=w470:u32)
                  n147 = Logical Shift(y=w465, x=w459) -> (x << y=w468:u32)
                  n148 = Logical Shift(y=w464, x=w459) -> (x << y=w469:u32)
                  n149 = And(x=w463, y=w470) -> (x .and. y?=w455:u32)
                  n150 = And(x=w460, y=w468) -> (x .and. y?=w454:u32)
                  n151 = And(x=w461, y=w469) -> (x .and. y?=w453:u32)
                  n152 = Type Cast(x=w455) -> (*(type *) &x=w458:string)  [unwired: 1 in]
                  n153 = Type Cast(x=w454) -> (*(type *) &x=w457:string)  [unwired: 1 in]
                  n154 = Type Cast(x=w453) -> (*(type *) &x=w456:string)  [unwired: 1 in]
                  n155 = Reverse String(1:w458) -> (0:w452:string)
                  n156 = Reverse String(1:w457) -> (0:w451:string)
                  n157 = Reverse String(1:w456) -> (0:w450:string)
                  n158 = Concatenate Strings(w452, w451, w450) -> (w449:string)
                  n159 = Concatenate Strings(w472, w449) -> (w448:string)
                  n160 = call "MD5.vi"("Message String"=w448) -> ("MD5 (16-bytes)"=w447:string)  [unwired: 9 in, 1 out]
                  n161 = Equal?(x=w471, y=w447) -> (x = y?=w462:bool)
                }
              }
            }
            n162 = Bundle By Name(cluster=w433, "Pswrd Salt (md5)"=w424) -> (w426:T5)
          }
          frame "get_diagram_heap" {
            # "Diagram (md5)"
            # "BDHP, BDHb, BDHc - Block Diagram Heap (Source Code)\nFPHP, FPHb, FPHc - Front Panel Heap (Source Code)"
            # "Block Diagram/Front Panel Heap (LabVIEW Version .. 5)\nBlock Diagram/Front Panel Heap Version B (LabVIEW Version 6 .. 9) - Compressed using deflate\nBlock Diagram/Front Panel Heap Version C (LabVIEW Version 10 .. 22) - Compressed using deflate"
            n163 = Unbundle By Name(w487) -> ("BDHx"=w486:i32)
            n164 = Index Array(array=w485, index=w486) -> (element=w484:T2)
            n165 = Unbundle By Name(w484) -> ("Name"=w478:string, "Data"=w479:string)
            n166 = Equal?(x=string[] ["BDHb", "BDHc", "FPHb", "FPHc"], y=w478) -> (x = y?=w482:bool[])
            n167 = Or Array Elements(Boolean array=w482) -> (logical OR=w481:bool)
            n168 = case "Is Compressed?" shown="True" w481 {
              tunnel: w479 -> [w493 w505]
              tunnel: w480 -> [w492 w500]
              tunnel: [w492 w496] -> w477
              tunnel: [w493 w494] -> w476
              frame False {
              }
              frame True {
                w502 = u32 0  # Uncompressed Size
                n169 = Unflatten From String(type=w502, binary string=w505, error in (no error)=w500) -> (rest of the binary string=w504:string, value=w501:u32, error out=w503:errorcluster)  [unwired: 2 in]
                n170 = call "zlib Uncompress.vi"("error in (no error)"=w503, "Uncompressed Size in"=w501, "Compressed Data in"=w504) -> ("error out"=w497:errorcluster, "Uncompressed Data out"=w495:string)  [unwired: 6 in, 1 out]
                n171 = Unflatten From String(type="", binary string=w495, data includes array or string size? (T)=TRUE, error in (no error)=w497) -> (value=w494:string, error out=w496:errorcluster)  [unwired: 1 in, 1 out]
              }
            }
            n172 = call "MD5.vi"("Message String"=w476) -> ("MD5 (16-bytes)"=w474:string)  [unwired: 9 in, 1 out]
            n173 = Bundle By Name(cluster=w488, "Diagram (md5)"=w474) -> (w475:T5)
          }
          frame "calc_new_password" {
            w522 = ""  # New Password ("")
            # "BDPW data"
            # "LVSR data"
            # "Replace BDPW"
            # "Hash2 (MD5)"
            # "Diagram (MD5)"
            # "Hash1 (MD5)"
            # "New Password (MD5)\nLIBN (delimiter ':')\nLVSR\n<Salt (MD5)>"
            # "Pwrd (MD5)"
            # "Pwrd (MD5)\nHash1 (MD5)\nHash2 (MD5)"
            n174 = Unbundle By Name(w521) -> ("Owning Libs (':')"=w520:string, "Pswrd Salt (md5)"=w519:string, "Diagram (md5)"=w518:string)
            n175 = Unbundle By Name(w517) -> ("BDPW"=w516:i32, "LVSR"=w513:i32)
            n176 = Index Array(array=w515, index #1=w516, index #2=w513) -> (element #1=w514:T2, element #2=w512:T2)
            n177 = Unbundle By Name(w512) -> ("Data"=w510:string)
            n178 = call "MD5.vi"("Message String"=w522) -> ("MD5 (16-bytes)"=w525:string)  [unwired: 9 in, 1 out]
            n179 = Concatenate Strings(w525, w520, w510, w519) -> (w527:string)
            n180 = call "MD5.vi"("Message String"=w527) -> ("MD5 (16-bytes)"=w524:string)  [unwired: 9 in, 1 out]
            n181 = Concatenate Strings(w524, w518) -> (w526:string)
            n182 = call "MD5.vi"("Message String"=w526) -> ("MD5 (16-bytes)"=w523:string)  [unwired: 9 in, 1 out]
            n183 = Unbundle By Name(w514) -> ("Offset"=w506:u32, "Data"=w511:string)
            n184 = Concatenate Strings(w525, w524, w523) -> (w528:string)
            n185 = Replace Substring(3:0 ("offset (0)"), 4:w528, 5:w511) -> (1:w508:string)  [unwired: 1 in, 1 out]
            n186 = Bundle By Name(cluster=w521, "BDPW Offset"=w506, "New BDPW"=w508) -> (w509:T5)
          }
          frame "new_vi" {
            # "Copy source VI and replace the BDPW block data, \nthen use VI scripting to create a clone of the VI\nto open in a new application context, finally delete\nthe temporary file."
            n187 = Unbundle By Name(w539) -> ("BDPW Offset"=w537:u32, "New BDPW"=w538:string)
            n188 = Read from Binary File(5:u8 0 ("unsigned byte array"), 8:w535, 10:-1 ("count (1)"), 11:w540) -> (0:w563:errorcluster, 2:w559:u8[], 3:w562:refnum<file>)  [unwired: 2 in, 1 out]
            n189 = String To Byte Array(string=w538) -> (unsigned byte array=w558:u8[])
            n190 = Close File(refnum=w562, error in=w563) -> (error out=w543:errorcluster)  [unwired: 1 out]
            n191 = Replace Array Subset(array=w559, new element=w558, index=w537) -> (w549:u8[])
            n192 = call <vilib>:"Get File Extension.vi"("error in (no error)"=w543, "file"=w540) -> ("error out"=w545:errorcluster, "filename without extension"=w544:string)  [unwired: 5 in, 3 out]
            n193 = call <vilib>:"Generate Temporary File Path.vi"("error in (no error)"=w545, "Temporary File Extension (tmp)"=w544) -> ("error out"=w542:errorcluster, "Unique Temporary File Path"=w550:path)  [unwired: 8 in]
            n194 = Open/Create/Replace File(file path (use dialog)=w550, error in=w542, operation (0:open)=T3."replace or create", access (0:read/write)=enum16{"read/write", "read-only", "write-only"}."write-only") -> (refnum out=w552:refnum<file>, error out=w555:errorcluster)  [unwired: 3 out]
            n195 = Write to Binary File(file (use dialog)=w552, data=w549, error in=w555, 5:FALSE ("prepend array or string size? (T)")) -> (refnum out=w554:refnum<file>, error out=w553:errorcluster)  [unwired: 2 in, 1 out]
            n196 = Close File(refnum=w554, error in=w553) -> (path=w547:path, error out=w548:errorcluster)
            n197 = case shown="No Error" w548 {
              selector: w548 -> [w577 w581]
              tunnel: [w578 w581] -> w546
              tunnel: w547 -> [w576 _]
              frame No Error {
                n198 = New VI(8:w577, 10:w576) -> (0:w580:errorcluster, 3:w575:refnum<vi>)  [unwired: 5 in]
                n199 = invoke class="VI" method="FP.Open"(reference=w575, error in=w580) -> (reference out=w573:refnum<vi>, error out=w579:errorcluster)  [unwired: 3 in, 3 out]
                n200 = invoke class="VI" method="Lock State.Set"(reference=w573, error in=w579, "lockState"=T7."Not Locked" ("Lock State")) -> (reference out=w572:refnum<vi>, error out=w574:errorcluster)  [unwired: 4 in, 5 out]
                n201 = Close Reference(reference=w572, error in (no error)=w574) -> (error out=w578:errorcluster)
              }
              frame Error {
              }
            }
            n202 = flat-sequence {
              tunnel: w547 -> [w570]
              tunnel: [w569] -> w536
              tunnel: w546 -> [w569]
              frame #0 {
                n203 = Delete(path (use dialog)=w570) -> ()  [unwired: 4 in, 3 out]
              }
            }
          }
        }
        n204 = Or(x=w20, y=w17) -> (x .or. y?=w19:bool)
      }
    }
    frame Error {
    }
  }
  "error out" <- w2
